vi "Handle dP dT.vi"(8 "error in (no error)":errorcluster, 11 "Stand in":refnum<class "Stand.lvclass">) -> (0 "error out":errorcluster, 3 "Stand out":refnum<class "Stand.lvclass">, 4 "dt ms":u32)   [LabVIEW 2019, in "Stand.lvclass"]
uses:
  Stand.lvclass
  Stand.lvclass/Stand.ctl
  dY_dX_Calculator/delayValue.lvclass/delayValue.ctl
  FPGA/TypeDef/AI index.ctl
  AI_class/AI.lvclass/AI.ctl
  AnalogComparator_class/AnalogComparator.lvclass/AnalogComparator.ctl
  d0b32f7e-a2eb-4dff-9ec3-f7480154de2a.vi
  AnalogComparator_class/GetStatus.vi
  <vilib>/Utility/error.llb/Clear Errors.vi
  dY_dX_Calculator/delayValue.lvclass
  AI_class/AI.lvclass
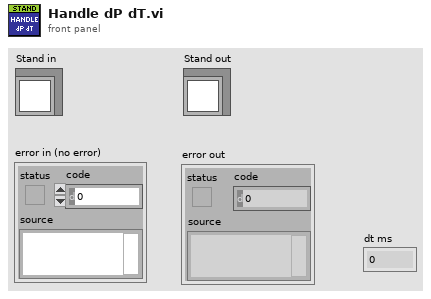
[diagram p1: front panel]
types:
  T1 = typedef "AI index.ctl" = u8
  T2 = typedef "AI_Data.ctl" = cluster{"Stat Data":T3, "OutOfRangeMax":bool, "OutOfRangeMin":bool, "HIHI":bool, "HI":bool, "LO":bool, "LOLO":bool}
  T3 = typedef "AI Statistics Data.ctl" = cluster{"raw mean":dbl, "scl mean":dbl, "raw mean 1Hz":dbl, "scl mean 1Hz":dbl}
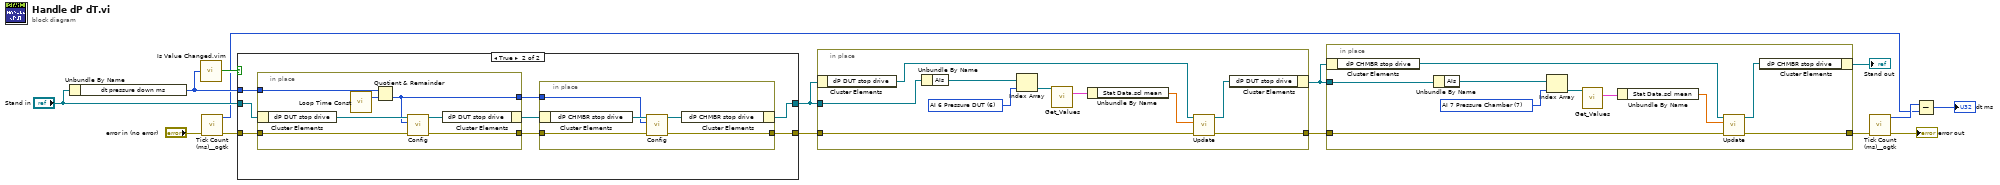
[diagram p0: block diagram]
diagram:
  n1 = Unbundle By Name("Stand in") -> ("dt pressure down ms"=w10:i32)
  n2 = call "Is Value Changed.vim"("value"=w10) -> ("changed or first call?"=w11:bool)
  n3 = call <userlib>:"Tick Count (ms)__ogtk.vi"("error in (no error)"="error in (no error)") -> ("error out"=w6:errorcluster, "millisecond timer value"=w2:u32)  [unwired: 9 in]
  n4 = case shown="True" w11 {
    tunnel: w6 -> [w16 w25]
    tunnel: "Stand in" -> [w17 w24]
    tunnel: w10 -> [_ w23]
    tunnel: [w17 w21] -> w12
    tunnel: [w16 w19] -> w13
    frame False {
    }
    frame True {
      n5 = in-place {
        in-place-border: w25 -> [w34]
        in-place-border: [w33] -> w20
        in-place-border: w23 -> [w32]
        in-place-border: [w31] -> w18
        n6 = in-place-cluster #1(w24) -> ("dP DUT stop drive"=w37:refnum<class "delayValue.lvclass">)
        n7 = call "Loop Time Const.vi"() -> ("loop time ms"=w35:i64)  [unwired: 3 in]
        n8 = Quotient & Remainder(x=w32, y=w35) -> (floor(x/y)=w31:i64)  [unwired: 1 out]
        n9 = call "Config.vi"("error in (no error)"=w34, "size (10)"=w31, "dY_dX_Calculator in"=w37) -> ("error out"=w33:errorcluster, "dY_dX_Calculator out"=w36:refnum<class "delayValue.lvclass">)  [unwired: 7 in]
        n10 = in-place-cluster #1("dP DUT stop drive"=w36) -> (w22:refnum<class "Stand.lvclass">)
      }
      n11 = in-place {
        in-place-border: w20 -> [w28]
        in-place-border: [w27] -> w19
        in-place-border: w18 -> [w26]
        n12 = in-place-cluster #2(w22) -> ("dP CHMBR stop drive"=w30:refnum<class "delayValue.lvclass">)
        n13 = call "Config.vi"("error in (no error)"=w28, "size (10)"=w26, "dY_dX_Calculator in"=w30) -> ("error out"=w27:errorcluster, "dY_dX_Calculator out"=w29:refnum<class "delayValue.lvclass">)  [unwired: 7 in]
        n14 = in-place-cluster #2("dP CHMBR stop drive"=w29) -> (w21:refnum<class "Stand.lvclass">)
      }
    }
  }
  n15 = in-place {
    in-place-border: w13 -> [w46]
    in-place-border: [w43] -> w8
    in-place-border: w12 -> [w39]
    w40 = T1 6 items=["AI 0 Cooling Station Level", "AI 1 Cooling Station Temp", "AI 2 Oil Supply Level", "AI 3 Oil Supply Temp", "AI 4 ", "AI 5 Pressure Haskel", "AI 6 Pressure DUT", "AI 7 Pressure Chamber", "AI 8 Pressure Air inlet", "AI 9 Pressure Air outlet", "AI 10 Pressure Messure Line"] ("AI index")
    n16 = in-place-cluster #3(w12) -> ("dP DUT stop drive"=w47:refnum<class "delayValue.lvclass">)
    n17 = Unbundle By Name(w39) -> ("AIs"=w41:refnum<class "AI.lvclass">[])
    n18 = Index Array(array=w41, index=w40) -> (element=w38:refnum<class "AI.lvclass">)
    n19 = call "Get_Values.vi"("reference in"=w38) -> ("Data"=w45:T2)  [unwired: 14 in]
    n20 = Unbundle By Name(w45) -> ("Stat Data.scl mean"=w44:dbl)
    n21 = call "Update.vi"("error in (no error)"=w46, "Value"=w44, "dY_dX_Calculator in"=w47) -> ("error out"=w43:errorcluster, "dY_dX_Calculator out"=w42:refnum<class "delayValue.lvclass">)  [unwired: 7 in]
    n22 = in-place-cluster #3("dP DUT stop drive"=w42) -> (w9:refnum<class "Stand.lvclass">)
  }
  n23 = in-place {
    in-place-border: w8 -> [w56]
    in-place-border: [w55] -> w5
    in-place-border: w9 -> [w49]
    w50 = T1 7 items=["AI 0 Cooling Station Level", "AI 1 Cooling Station Temp", "AI 2 Oil Supply Level", "AI 3 Oil Supply Temp", "AI 4 ", "AI 5 Pressure Haskel", "AI 6 Pressure DUT", "AI 7 Pressure Chamber", "AI 8 Pressure Air inlet", "AI 9 Pressure Air outlet", "AI 10 Pressure Messure Line"] ("AI index")
    n24 = in-place-cluster #4(w9) -> ("dP CHMBR stop drive"=w57:refnum<class "delayValue.lvclass">)
    n25 = Unbundle By Name(w49) -> ("AIs"=w51:refnum<class "AI.lvclass">[])
    n26 = Index Array(array=w51, index=w50) -> (element=w48:refnum<class "AI.lvclass">)
    n27 = call "Get_Values.vi"("reference in"=w48) -> ("Data"=w54:T2)  [unwired: 14 in]
    n28 = Unbundle By Name(w54) -> ("Stat Data.scl mean"=w53:dbl)
    n29 = call "Update.vi"("error in (no error)"=w56, "Value"=w53, "dY_dX_Calculator in"=w57) -> ("error out"=w55:errorcluster, "dY_dX_Calculator out"=w52:refnum<class "delayValue.lvclass">)  [unwired: 7 in]
    n30 = in-place-cluster #4("dP CHMBR stop drive"=w52) -> (→"Stand out":refnum<class "Stand.lvclass">)
  }
  n31 = call <userlib>:"Tick Count (ms)__ogtk.vi"("error in (no error)"=w5) -> ("error out"=→"error out":errorcluster, "millisecond timer value"=w3:u32)  [unwired: 9 in]
  n32 = Subtract(x=w3, y=w2) -> (x-y=→"dt ms":u32)
